vi "Motor Control NO PID.vi"(2 "error in (no error)":errorcluster, 3 "Yaw":dbl, 4 "Speed":dbl, 5 "Direction":T1) -> (0 "error out":errorcluster, 1 "Speed & distance":T2)   [LabVIEW 2018]
uses:
  MOTOR CONTROL NO PID Type Def.ctl
  <vilib>/Studica/Studica Toolkit/Background/Mxp Selection.ctl
panel:
  out "M2":dbl
  out "M1":dbl
  out "M0":dbl
  out "S2":dbl
  out "S1":dbl
  out "S0":dbl
  out "M2 Distance":dbl
  out "M1 Distance":dbl
  out "M0 Distance":dbl
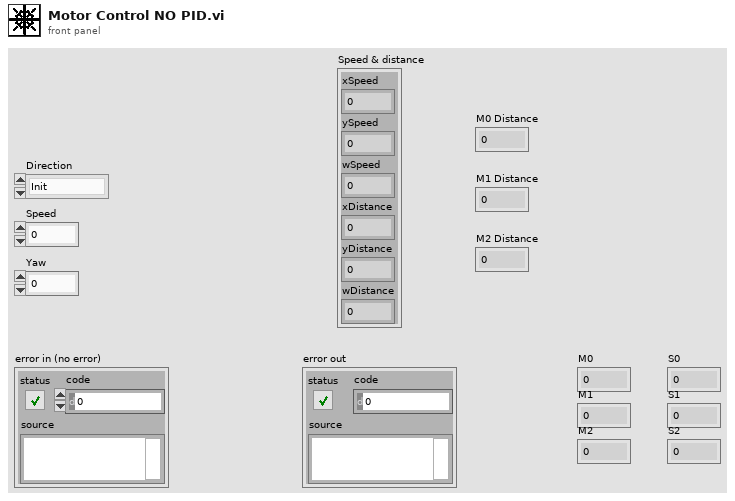
[diagram p1: front panel]
types:
  T1 = typedef "MOTOR CONTROL NO PID Type Def.ctl" = enum16{"Init", "Front Back", "Left Right", "Rotate", "Stop", "Latch"}
  T2 = cluster{"xSpeed":dbl, "ySpeed":dbl, "wSpeed":dbl, "xDistance":dbl, "yDistance":dbl, "wDistance":dbl}
  T3 = typedef "Mxp Selection.ctl" = enum16{"MXP A", "MXP B"}
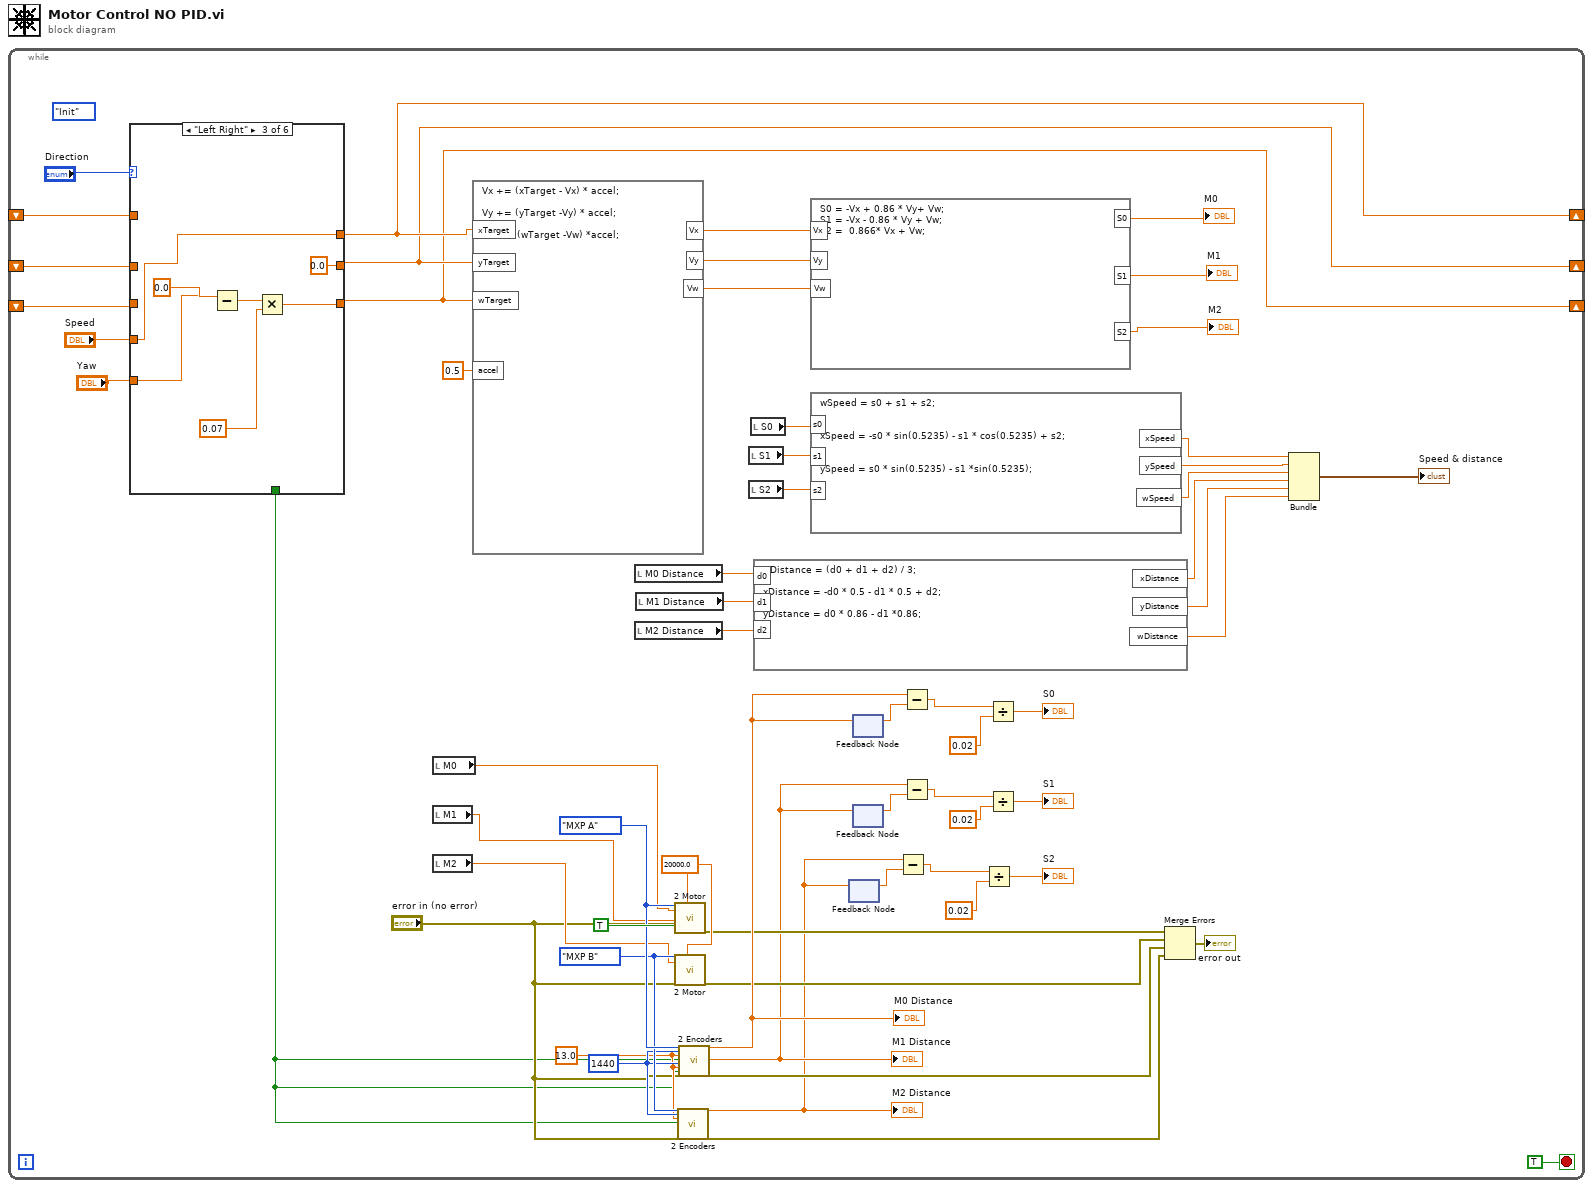
[diagram p0: block diagram]
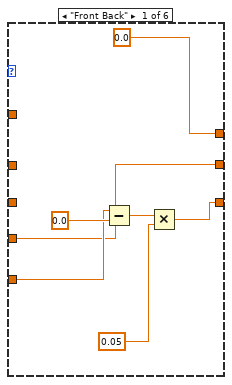
[diagram p2: hidden frame]
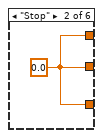
[diagram p3: hidden frame]
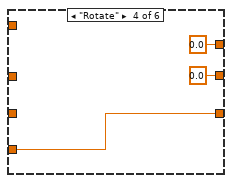
[diagram p4: hidden frame]
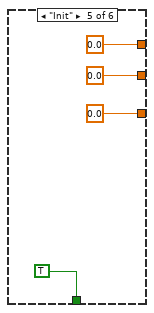
[diagram p5: hidden frame]
diagram:
  n1 = while {
    shift-right: [w4] -> _
    shift-left: _ -> [w7]
    shift-right: [w3] -> _
    shift-left: _ -> [w6]
    shift-right: [w2] -> _
    shift-left: _ -> [w5]
    stop <- TRUE stop-if-true
    (unwired) MOTOR_CONTROL_NO_PID_Type_Def."Init" ("Direction")
    w56 = 13.0 ("Wheel Diameter M0 (inches)")
    w57 = u32 1440 ("Ticks Per Rev M0")
    w61 = 20000.0 ("Frequency [Hz]")
    w59 = Mxp_Selection."MXP A" ("Mxp Side")
    w58 = Mxp_Selection."MXP B" ("Mxp Side")
    n2 = case shown="\"Left Right\"" "Direction" {
      tunnel: [0.0 w69 w76 0.0 ("Speed") 0.0 w86] -> w4
      tunnel: [w62 w69 0.0 ("Speed") 0.0 ("Speed") 0.0 w85] -> w3
      tunnel: [w64 w69 w71 w77 0.0 w84] -> w2
      tunnel: "Speed" -> [w62 _ w76 w77 _ _]
      tunnel: "Yaw" -> [w63 _ w70 _ _ _]
      tunnel: [_ _ _ _ TRUE ("Invert M1") _] -> w12
      tunnel: w7 -> [_ _ _ _ _ w86]
      tunnel: w6 -> [_ _ _ _ _ w85]
      tunnel: w5 -> [_ _ _ _ _ w84]
      frame "Front Back" {
        n3 = Subtract(x=w63, y=0.0) -> (x-y=w67:dbl)
        n4 = Multiply(x=w67, y=0.05) -> (x*y=w64:dbl)
      }
      frame "Stop" {
        w69 = 0.0
      }
      frame "Left Right" {
        n5 = Subtract(x=w70, y=0.0) -> (x-y=w74:dbl)
        n6 = Multiply(x=w74, y=0.07) -> (x*y=w71:dbl)
      }
      frame "Rotate" {
      }
      frame "Init" {
      }
      frame "Latch", Default {
      }
    }
    n7 = local read "M0"() -> (w35:dbl)
    n8 = local read "M1"() -> (w34:dbl)
    n9 = local read "M2"() -> (w33:dbl)
    n10 = formula code="Vx += (xTarget - Vx) * accel;\n\nVy += (yTarget -Vy) * accel;\n\nVw += (wTarget -Vw) *accel;"("xTarget"=w4, "yTarget"=w3, "wTarget"=w2, "accel"=0.5 ("input variable")) -> ("Vy"=w14:dbl, "Vx"=w15:dbl, "Vw"=w13:dbl)
    n11 = local read "M0 Distance"() -> (w29:dbl)
    n12 = local read "M2 Distance"() -> (w27:dbl)
    n13 = local read "M1 Distance"() -> (w28:dbl)
    n14 = call <vilib>:"2 Motor.vi"("Mxp Side"=w59, "Speed M0"=w35, "Speed M1"=w34, "Invert M1"=TRUE, "error in (no error)"="error in (no error)", "Frequency [Hz]"=w61) -> ("error out"=w51:errorcluster)  [unwired: 13 in]
    n15 = call <vilib>:"2 Motor.vi"("Mxp Side"=w58, "Speed M0"=w33, "error in (no error)"="error in (no error)", "Frequency [Hz]"=w61) -> ("error out"=w50:errorcluster)  [unwired: 15 in]
    n16 = call <vilib>:"2 Encoders.vi"("Mxp Side"=w58, "Ticks Per Rev M0"=w57, "Wheel Diameter M0 (inches)"=w56, "Reset Encoder 0"=w12, "error in (no error)"="error in (no error)") -> ("Distance M0 (inches)"=w39:dbl, "error out"=w48:errorcluster)  [unwired: 20 in, 1 out]
    "M2 Distance" <- w39
    n17 = call <vilib>:"2 Encoders.vi"("Mxp Side"=w59, "Ticks Per Rev M0"=w57, "Wheel Diameter M0 (inches)"=w56, "Reset Encoder 0"=w12, "Ticks Per Rev M1"=w57, "Wheel Diameter M1 (inches)"=w56, "Reset Encoder 1"=w12, "error in (no error)"="error in (no error)") -> ("Distance M0 (inches)"=w54:dbl, "Distance M1 (inches)"=w43:dbl, "error out"=w49:errorcluster)  [unwired: 17 in]
    "M0 Distance" <- w54
    "M1 Distance" <- w43
    n18 = local read "S1"() -> (w31:dbl)
    n19 = local read "S2"() -> (w30:dbl)
    n20 = local read "S0"() -> (w32:dbl)
    n21 = formula code="wDistance = (d0 + d1 + d2) / 3;\n\nxDistance = -d0 * 0.5 - d1 * 0.5 + d2;\n\nyDistance = d0 * 0.86 - d1 *0.86;"("d0"=w29, "d1"=w28, "d2"=w27) -> ("xDistance"=w22:dbl, "wDistance"=w20:dbl, "yDistance"=w21:dbl)
    n22 = formula code="S0 = -Vx + 0.86 * Vy+ Vw;\nS1 = -Vx - 0.86 * Vy + Vw;\nS2 =  0.866* Vx + Vw;"("Vx"=w15, "Vy"=w14, "Vw"=w13) -> ("S0"=→"M0":dbl, "S1"=→"M1":dbl, "S2"=→"M2":dbl)
    n23 = formula code="wSpeed = s0 + s1 + s2;\n\n\nxSpeed = -s0 * sin(0.5235) - s1 * cos(0.5235) + s2;\n\n\nySpeed = s0 * sin(0.5235) - s1 *sin(0.5235);"("s0"=w32, "s1"=w31, "s2"=w30) -> ("xSpeed"=w26:dbl, "ySpeed"=w25:dbl, "wSpeed"=w24:dbl)
    n24 = feedback #1() -> (w41:dbl)  [unwired: 1 in]
    n25 = feedback-in #1(w39) -> ()
    n26 = feedback #2() -> (w53:dbl)  [unwired: 1 in]
    n27 = feedback-in #2(w54) -> ()
    n28 = feedback #3() -> (w45:dbl)  [unwired: 1 in]
    n29 = feedback-in #3(w43) -> ()
    n30 = Subtract(x=w39, y=w41) -> (x-y=w42:dbl)
    n31 = Subtract(x=w54, y=w53) -> (x-y=w55:dbl)
    n32 = Subtract(x=w43, y=w45) -> (x-y=w46:dbl)
    n33 = Divide(x=w42, y=0.02) -> (x/y=→"S2":dbl)
    n34 = Divide(x=w55, y=0.02) -> (x/y=→"S0":dbl)
    n35 = Divide(x=w46, y=0.02) -> (x/y=→"S1":dbl)
    n36 = Merge Errors(w51, w50, w49, w48) -> (→"error out":errorcluster)
    n37 = Bundle("xSpeed"=w26, "ySpeed"=w25, "wSpeed"=w24, "xDistance"=w22, "yDistance"=w21, "wDistance"=w20) -> (→"Speed & distance":T2)  [unwired: 1 in]
  }
